vi "Popup Message.vi"(1 "Seconds to display":u32) -> ()   [LabVIEW 2016]
uses:
  Types/Global Variables.vi
panel:
  out "Message\nDisplayed":string
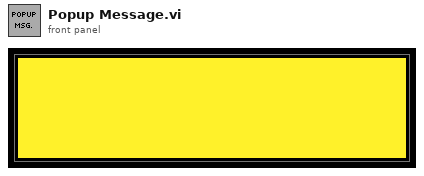
[diagram p1: front panel]
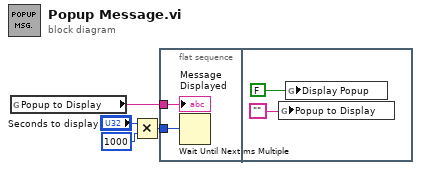
[diagram p0: block diagram]
diagram:
  n1 = global read "Global Variables.vi" "Popup to Display"() -> (w1:string)
  n2 = Multiply(x="Seconds to display", y=u32 1000) -> (x*y=w3:u32)
  n3 = flat-sequence {
    tunnel: w1 -> [w6]
    tunnel: w3 -> [w5]
    frame #0 {
      n4 = Wait Until Next ms Multiple(millisecond multiple=w5) -> ()  [unwired: 1 out]
      "Message\nDisplayed" <- w6
    }
    frame #1 {
      n5 = global write "Global Variables.vi" "Popup to Display"("") -> ()
      n6 = global write "Global Variables.vi" "Display Popup"(FALSE ("Display Popup")) -> ()
    }
  }
